vi "COM_W_R_Termination-ETX.vi"(0 "VISA resource name":refnum<visa-resource-name>="COM74", 1 "baud rate":u32=115200, 2 "data bits":u16=8 min=5 max=8 step=1, 3 "parity":u16(ring) items=["None", "Odd", "Even", "Mark", "Space"], 4 "stop bits":u16(ring)=10 items=["1.0"=10, "1.5"=15, "2.0"=20], 5 "write":bool=TRUE, 6 "read":bool=TRUE, 7 "flow control":u16(ring) items=["None"=0, "XON/XOFF"=1, "RTS/CTS"=2, "DTR/DSR"=4], 8 "string to write":string="*IDN?") -> (9 "read string":string, 10 "return count":u32)   [LabVIEW 2012]
doc: "The Basic Serial Read and Write example performs a Serial Port Read, a Serial Port Write, or a combination of these actions. The user selects the actions (read or write) on the front panel. If both are selected, the VI will write the data first, read data, and then close the VISA session that is opened to the port. This VI will wait until the specified number of bytes is received at the port. Only the number of bytes specified will be read.\n\nINSTRUCTIONS:\n1) Select the serial resource and configuration parameters (baud rate, data bits, parity, stop bits, flow control).\n2) Select the operations to be performed. \n3) Connect the serial port to your device. If no device is available, perform a loopback test by doing one of the following. Short pins 2 and 3 on a RS-232 cable or short pin 4 to pin 8 and pin 5 to pin 9 on a RS-485/422 cable. \n4) Run the VI to see the data read. (The \"read string\" will match the \"string to write\" if a loopback test was performed.)\n\nNote: The parameters set for the serial port must match the parameters of the connected instrument or device. In this example, the bytes to read parameter specifies the number of bytes that the serial port reads. If there were more bytes at the port than the number specified in bytes to read, those bytes would not be read. Also, if you specify to read more bytes than the number of bytes actually read, you might receive a timeout error message.\n\nOn the block diagram, the Configure Serial Port VI sets the configuration parameters. The front panel displays the controls used to configure the basic parameters, such as baud rate, data bits, and parity. Constants configure the other parameters the user probably does not need set. After the VISA Configure Serial Port VI opens the VISA session and configures the port, the VI passes the VISA resource name to other VIs that perform operations on that VISA resource. The VISA Write function sends a command to the serial device and the VISA Read function returns data based on the command. The VISA Close function then closes the reference to the serial device. It is important to close the reference; otherwise communication through with that port through protocols other than VISA might not be possible."
uses:
  <vilib>/Instr/_visa.llb/VISA Configure Serial Port (Instr).vi
panel:
  out "Bytes at Port":u32
  # "Select the serial resource and the operations (Read, Write, or both) to be performed.  If both are selected, the VI will write the data first, read data and then close the VISA session that is opened to the port.  This VI will wait until the specified number of bytes is received at the port. Only the number of bytes specified will be read."
  # "For additional information select File >> VI Properties >> Documentation"
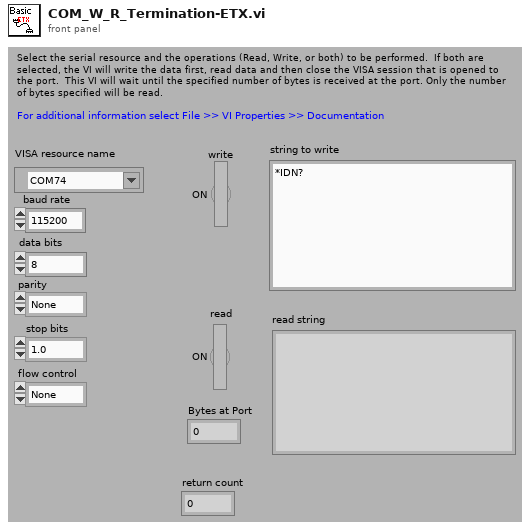
[diagram p1: front panel]
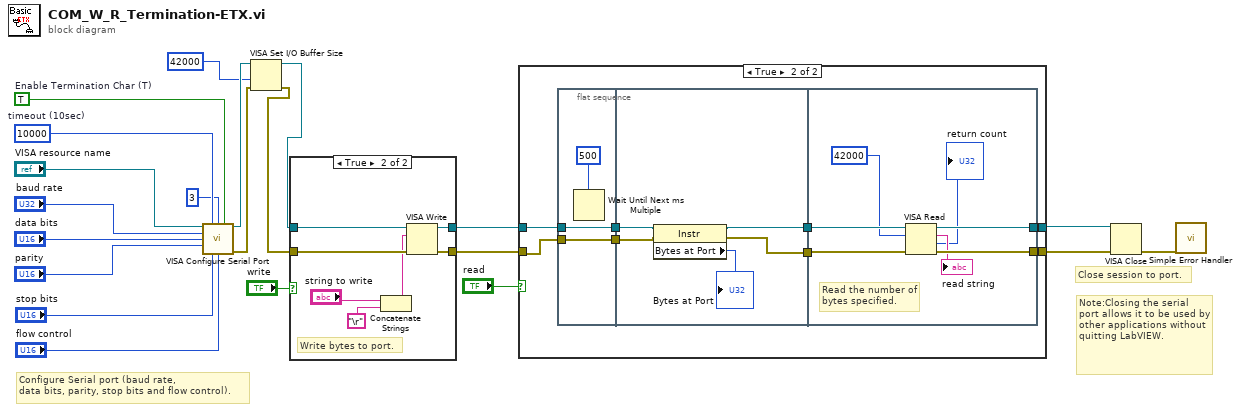
[diagram p0: block diagram]
diagram:
  w13 = TRUE  # Enable Termination Char (T)
  w14 = u32 10000  # timeout (10sec)
  # "Note:Closing the serial port allows it to be used by other applications without\nquitting LabVIEW."
  # "Configure Serial port (baud rate,\ndata bits, parity, stop bits and flow control)."
  # "Close session to port."
  n1 = call-poly "VISA Configure Serial Port"("VISA resource name"="VISA resource name", "timeout (10sec)"=w14, "termination char\n(0xA = '\\n' = LF)"=u8 3 ("termination char\n(0xA = '\\n' = LF)"), "Enable Termination\nChar (T)"=w13, "baud rate (9600)"="baud rate", "data bits (8)"="data bits", "parity (0:none)"="parity", "stop bits (10: 1 bit)"="stop bits", "flow control (0:none)"="flow control") -> ("VISA resource name out"=w5:refnum<visa-resource-name>, "error out"=w2:errorcluster)  [unwired: 5 in]
  n2 = VISA Set I/O Buffer Size(VISA resource name=w5, size (4096)=u32 42000, error in (no error)=w2) -> (VISA resource name out=w3:refnum<visa-resource-name>, error out=w1:errorcluster)  [unwired: 1 in]
  n3 = case shown="True" "write" {
    tunnel: [w23 w30] -> w19
    tunnel: w3 -> [w22 w29]
    tunnel: w1 -> [w23 w28]
    tunnel: [w22 w27] -> w9
    frame False {
    }
    frame True {
      # "Write bytes to port."
      n4 = Concatenate Strings("string to write", "\r") -> (w24:string)
      n5 = VISA Write(VISA resource name=w29, write buffer=w24, error in (no error)=w28) -> (VISA resource name out=w27:refnum<visa-resource-name>, error out=w30:errorcluster)  [unwired: 1 out]
    }
  }
  n6 = case shown="True" "read" {
    tunnel: w19 -> [w32 w37]
    tunnel: [w32 w40] -> w18
    tunnel: [w31 w39] -> w17
    tunnel: w9 -> [w31 w38]
    frame False {
    }
    frame True {
      n7 = flat-sequence {
        tunnel: w37 -> [w41]
        tunnel: w38 -> [w43]
        tunnel: [w43] -> w35
        tunnel: [w41] -> w34
        tunnel: [w44] -> w36
        tunnel: w35 -> [w47]
        tunnel: w34 -> [w46]
        tunnel: [w45] -> w33
        tunnel: [w55] -> w40
        tunnel: [w54] -> w39
        tunnel: w36 -> [w52]
        tunnel: w33 -> [w51]
        frame #0 {
          n8 = Wait Until Next ms Multiple(millisecond multiple=u32 500) -> ()  [unwired: 1 out]
        }
        frame #1 {
          n9 = property class="Instr"(reference=w47, error in=w46) -> (reference out=w44:refnum<visa-resource-name>, error out=w45:errorcluster, "Bytes at Port"=→"Bytes at Port":u32)
        }
        frame #2 {
          # "Read the number of bytes specified."
          n10 = VISA Read(VISA resource name=w52, byte count=u32 42000, error in (no error)=w51) -> (VISA resource name out=w54:refnum<visa-resource-name>, read buffer=→"read string":string, return count=→"return count":u32, error out=w55:errorcluster)
        }
      }
    }
  }
  n11 = VISA Close(VISA resource name=w17, error in (no error)=w18) -> (error out=w16:errorcluster)
  n12 = call <vilib>:"Simple Error Handler.vi"("error in (no error)"=w16) -> ()  [unwired: 4 in, 5 out]
